vi "Practica_6_Producto_Punto_Matriz_Matriz.vi"() -> ()   [LabVIEW 2016]
panel:
  out "Vector A 2":dbl[][](array[numeric])
  in  "Matriz B":dbl[][](array[numeric])
  in  "Matriz B":dbl[][](array[numeric])
  # "Practica #6 : Producto Punto Matriz Matriz"
  # "Resultado"
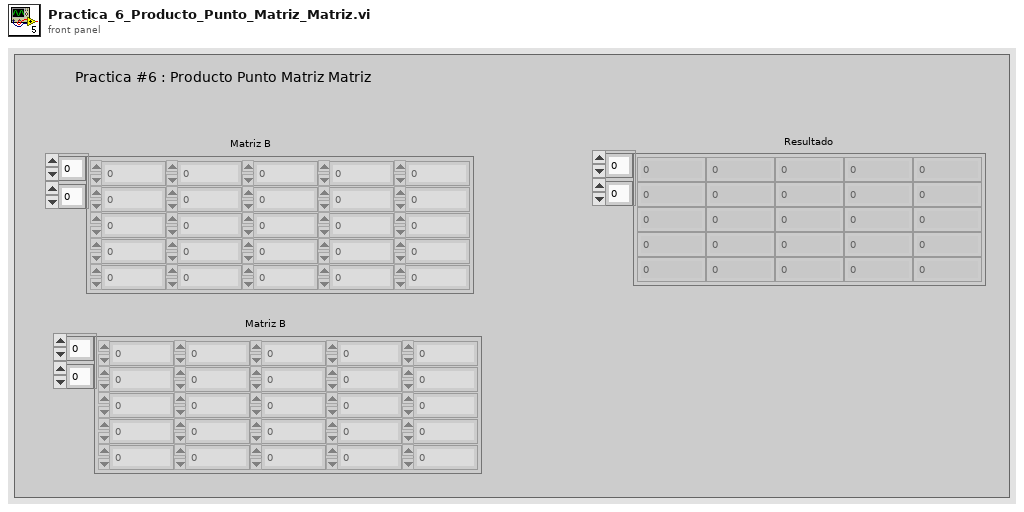
[diagram p1: front panel]
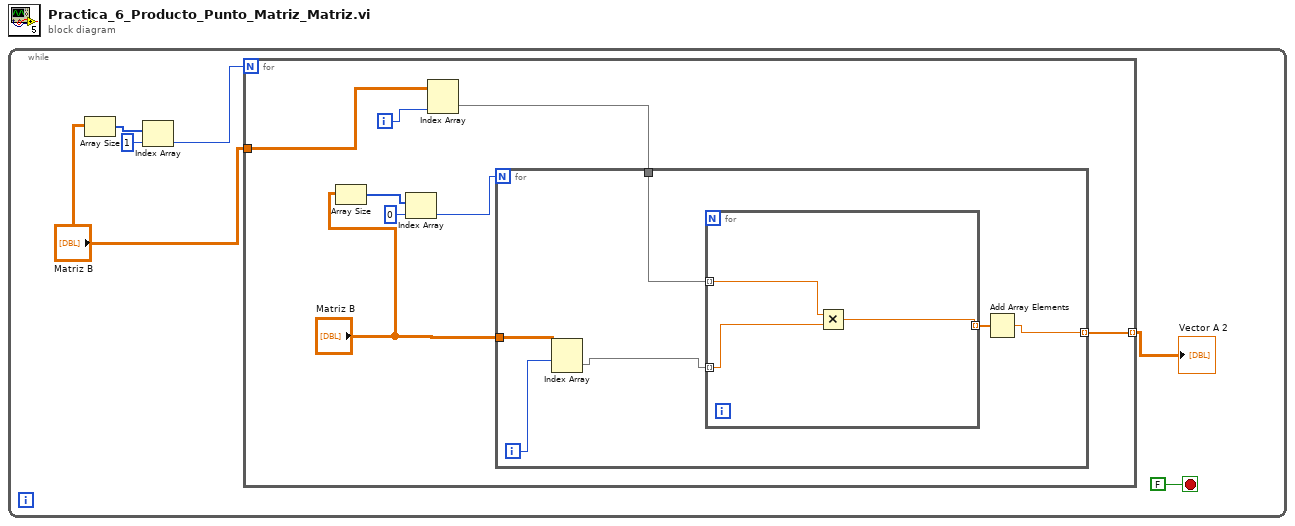
[diagram p0: block diagram]
diagram:
  n1 = while {
    stop <- FALSE stop-if-true
    n2 = Array Size(array="Matriz B") -> (size(s)=w4:i32[])
    n3 = Index Array(array=w4, index=1) -> (element=w3:i32)
    n4 = for {
      N: w3 -> [_]
      tunnel: [w14] -> w5 mode=indexing
      tunnel: "Matriz B" -> [w9]
      i -> [w8]
      n5 = Array Size(array="Matriz B") -> (size(s)=w13:i32[])
      n6 = Index Array(array=w13, index=0) -> (element=w12:i32)
      n7 = Index Array(array=w9, index (col)=w8) -> (element=w7:dbl[])  [unwired: 1 in]
      n8 = for {
        N: w12 -> [_]
        tunnel: "Matriz B" -> [w19]
        tunnel: [w16] -> w14 mode=indexing
        tunnel: w7 -> [w15]
        i -> [w18]
        n9 = Index Array(array=w19, index (row)=w18) -> (element=w17:dbl[])  [unwired: 1 in]
        n10 = for {
          tunnel: w17 -> [w23] mode=indexing
          tunnel: w15 -> [w22] mode=indexing
          tunnel: [w21] -> w20 mode=indexing
          n11 = Multiply(x=w22, y=w23) -> (x*y=w21:dbl)
        }
        n12 = Add Array Elements(numeric array=w20) -> (sum=w16:dbl)
      }
    }
    "Vector A 2" <- w5
  }
